vi "analysis_logging_data.vi"() -> ()   [LabVIEW 2020]
uses:
  <vilib>/Utility/file.llb/Read Delimited Spreadsheet (string).vi
panel:
  in  "Act_file_path":path=path "E:/Workspace/LabVIEW/Air_Flow_Meter_OCR/logging_data/program/Test-2020-12-15-오후-04-14-55.csv"
  in  "Ref_file_path":path=path "E:/Workspace/LabVIEW/Air_Flow_Meter_OCR/logging_data/program/Test-2020-12-15-오후-04-14-55.csv"
  out "Waveform Graph":i32[](graph)
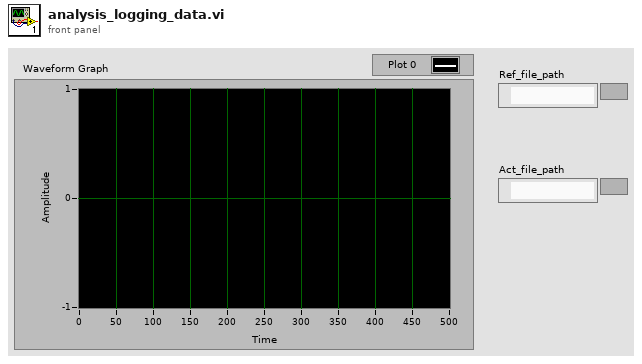
[diagram p1: front panel]
types:
  T1 = typedef "LVDateTimeRec.ctl" = cluster{"fractional second":dbl, "second":i32, "minute":i32, "hour":i32, "day of month":i32, "month":i32, "year":i32, "day of week":i32, "day of year":i32, "DST":i32}
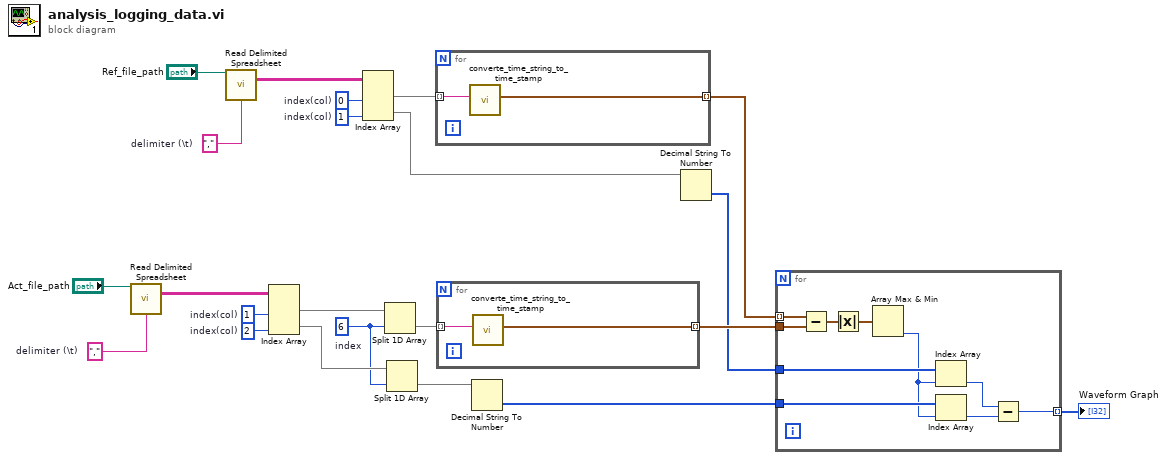
[diagram p0: block diagram]
diagram:
  w10 = 1  # index(col)
  w9 = 0  # index(col)
  w12 = ","  # delimiter (\t)
  w17 = 2  # index(col)
  w15 = 6  # index
  w19 = 1  # index(col)
  w21 = ","  # delimiter (\t)
  n1 = call-poly <vilib>:"Read Delimited Spreadsheet.vi"("file path (dialog if empty)"="Act_file_path", "delimiter (\\t)"=w21) -> ("all rows"=w20:string[][])  [unwired: 8 in, 5 out]
  n2 = call-poly <vilib>:"Read Delimited Spreadsheet.vi"("file path (dialog if empty)"="Ref_file_path", "delimiter (\\t)"=w12) -> ("all rows"=w8:string[][])  [unwired: 8 in, 5 out]
  n3 = Index Array(array=w20, index (col) #1=w19, index (col) #2=w17) -> (element #1=w18:string[], element #2=w16:string[])  [unwired: 2 in]
  n4 = Index Array(array=w8, index (col) #1=w9, index (col) #2=w10) -> (element #1=w5:string[], element #2=w4:string[])  [unwired: 2 in]
  n5 = Split 1D Array(array=w18, index=w15) -> (second subarray=w7:string[])  [unwired: 1 out]
  n6 = Split 1D Array(array=w16, index=w15) -> (second subarray=w14:string[])  [unwired: 1 out]
  n7 = for {
    tunnel: w5 -> [w24] mode=indexing
    tunnel: [w23] -> w1 mode=indexing
    n8 = call "converte_time_string_to_time_stamp.vi"("input_string"=w24) -> ("date time rec"=w23:T1)  [unwired: 10 in]
  }
  n9 = for {
    tunnel: w7 -> [w26] mode=indexing
    tunnel: [w25] -> w6 mode=indexing
    n10 = call "converte_time_string_to_time_stamp.vi"("input_string"=w26) -> ("date time rec"=w25:T1)  [unwired: 10 in]
  }
  n11 = Decimal String To Number(string=w14) -> (number=w13:i32[])  [unwired: 2 in, 1 out]
  n12 = Decimal String To Number(string=w4) -> (number=w3:i32[])  [unwired: 2 in, 1 out]
  n13 = for {
    tunnel: w13 -> [w28]
    tunnel: w6 -> [w31]
    tunnel: w1 -> [w29] mode=indexing
    tunnel: w3 -> [w34]
    tunnel: [w30] -> w2 mode=indexing
    n14 = Subtract(x=w29, y=w31) -> (x-y=w36:T1[])
    n15 = Absolute Value(x=w36) -> (abs(x)=w35:T1[])
    n16 = Array Max & Min(array=w35) -> (min index (indices)=w27:i32)  [unwired: 3 out]
    n17 = Index Array(array=w34, index=w27) -> (element=w32:i32)
    n18 = Index Array(array=w28, index=w27) -> (element=w33:i32)
    n19 = Subtract(x=w32, y=w33) -> (x-y=w30:i32)
  }
  "Waveform Graph" <- w2
